vi "Util Hex String to U8 Array.vi"(8 "error in (no error)":errorcluster, 10 "Initial Offset":u32, 11 "Hex String":string) -> (0 "error out":errorcluster, 3 "U8 Array":u8[](array[numeric]) format="%x")   [LabVIEW 2017, in "xHelper.lvlib"]
uses:
  xHelper.lvlib
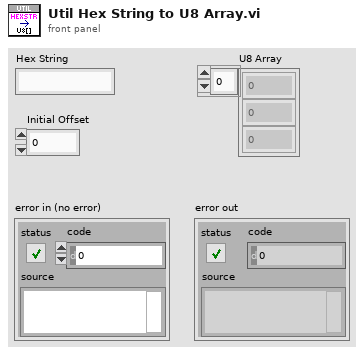
[diagram p1: front panel]
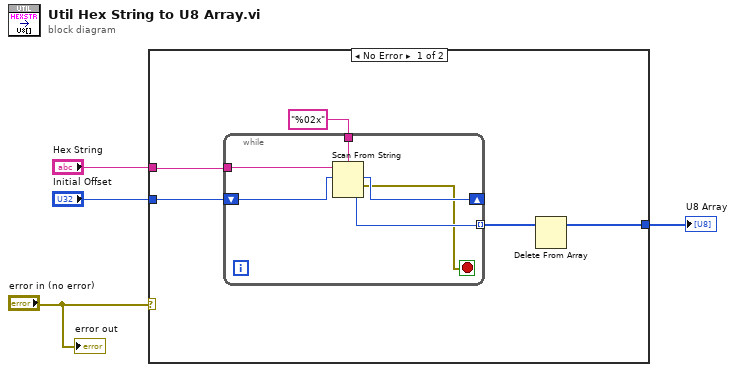
[diagram p0: block diagram]
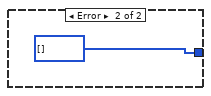
[diagram p2: hidden frame]
diagram:
  n1 = case shown="No Error" "error in (no error)" {
    tunnel: "Hex String" -> [w5 _]
    tunnel: "Initial Offset" -> [w7 _]
    tunnel: [w6 u32[] []] -> w1
    frame No Error {
      n2 = while {
        shift-right: [w13] -> _
        shift-left: w7 -> [w14]
        tunnel: "%02x" ("format string") -> [w15]
        tunnel: [w12] -> w9 mode=indexing
        tunnel: w5 -> [w10]
        stop <- w11 stop-if-true
        n3 = Scan From String(format string=w15, input string=w10, initial scan location=w14) -> (offset past scan=w13:u32, error out=w11:errorcluster, output 1=w12:u32)  [unwired: 2 in, 1 out]
      }
      n4 = Delete From Array "Delete From Array"(array=w9) -> (array with subset deleted=w6:u32[])  [unwired: 2 in, 1 out]
    }
    frame Error {
    }
  }
  "U8 Array" <- w1
  "error out" <- "error in (no error)"
